vi "Generate call result event.vi"(8 "error in (no error)":errorcluster, 10 "ICallResult":refnum<class "ICallResult.lvclass">, 11 "Events in":refnum<class "Events.lvclass">) -> (0 "error out":errorcluster, 3 "Events out":refnum<class "Events.lvclass">)   [LabVIEW 2020, in "wamplv.lvlib" / "Events.lvclass"]
uses:
  Events.lvclass
  Events.lvclass/Events.ctl
  Requests/Call/ICallResult/ICallResult.lvclass
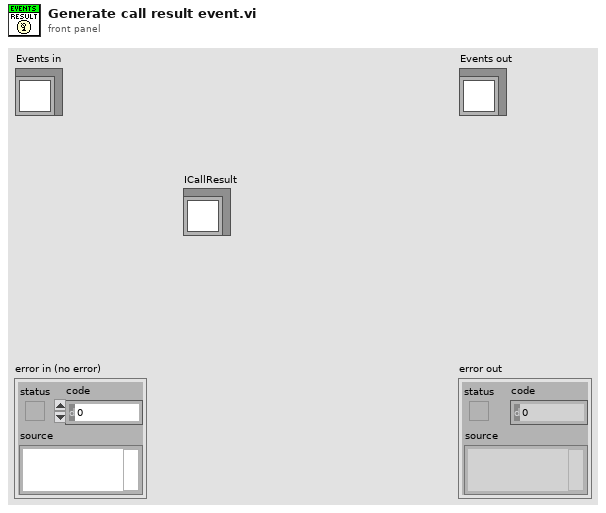
[diagram p1: front panel]
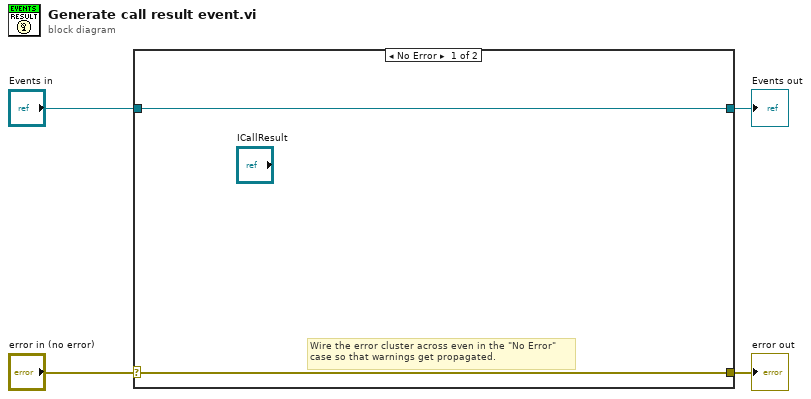
[diagram p0: block diagram]
diagram:
  n1 = case shown="No Error" "error in (no error)" {
    selector: "error in (no error)" -> [w5 w8]
    tunnel: [w5 w8] -> w3
    tunnel: [w6 w7] -> w1
    tunnel: "Events in" -> [w6 w7]
    frame No Error {
      # "Wire the error cluster across even in the \"No Error\"\ncase so that warnings get propagated."
    }
    frame Error {
    }
  }
  "error out" <- w3
  "Events out" <- w1
